vi "Plugin - Compute Turns.vi"(11 "Message Queues in":T1) -> ()   [LabVIEW 2019]
uses:
  support/Copy of Message Queue/All Message Queues.ctl
  support/Copy of Message Queue/Message Cluster.ctl
  support/Global Offsets.vi
  Acquisition/Acquisition.lvlib
  support/Message Queue/Message Queue.lvlib
  support/Copy of Message Queue/Copy of Message Queue.lvlib
panel:
  in  "OK":bool
  out "Turns Clockwise":dbl format="%.3f"
  in  "Stop":bool
  out "T12":dbl(slide) scale=0.0..30.0
  out "T11":dbl(slide) scale=0.0..30.0
  out "T10":dbl(slide) scale=0.0..30.0
  out "T9":dbl(slide) scale=0.0..30.0
  out "T8":dbl(slide) scale=0.0..30.0
  out "T7":dbl(slide) scale=0.0..30.0
  out "T6":dbl(slide) scale=0.0..30.0
  out "T5":dbl(slide) scale=0.0..30.0
  out "T4":dbl(slide) scale=0.0..30.0
  out "T3":dbl(slide) scale=0.0..30.0
  out "T2":dbl(slide) scale=0.0..30.0
  out "T1":dbl(slide) scale=0.0..30.0
  out "Aquatrak RS232 Output":string
  in  "error in":errorcluster
  out "error out":errorcluster
  # "Compute Turns Clockwise"
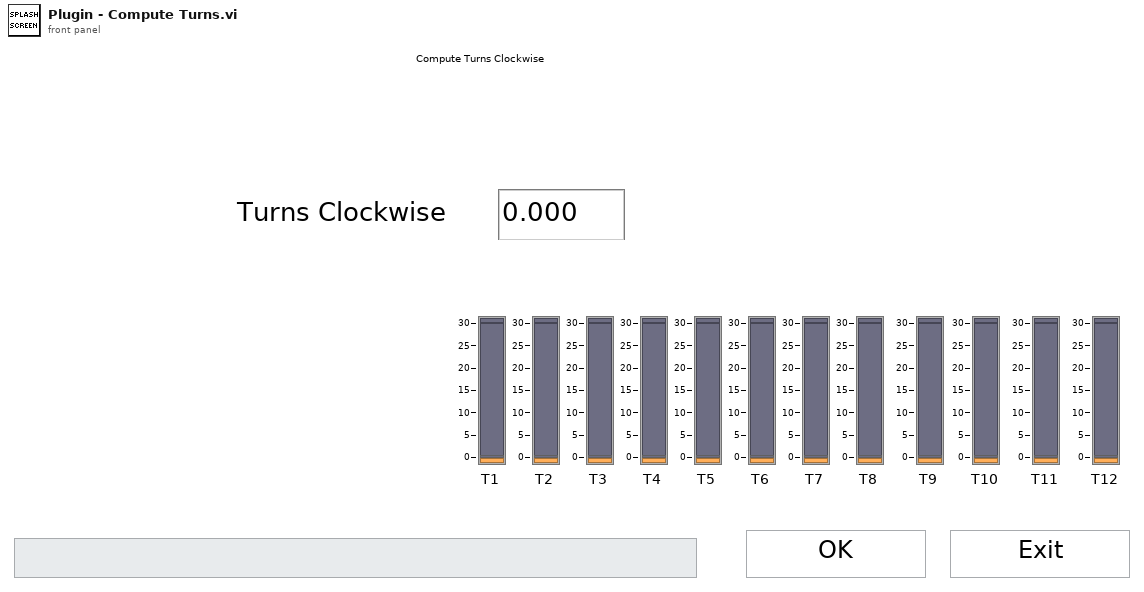
[diagram p1: front panel]
types:
  T1 = typedef "Copy of Message Queue.lvlib/All Message Queues.ctl" = cluster{"UI":refnum<queue>, "Acquisition":refnum<queue>, "Logging":refnum<queue>, "Analyze":refnum<queue>}
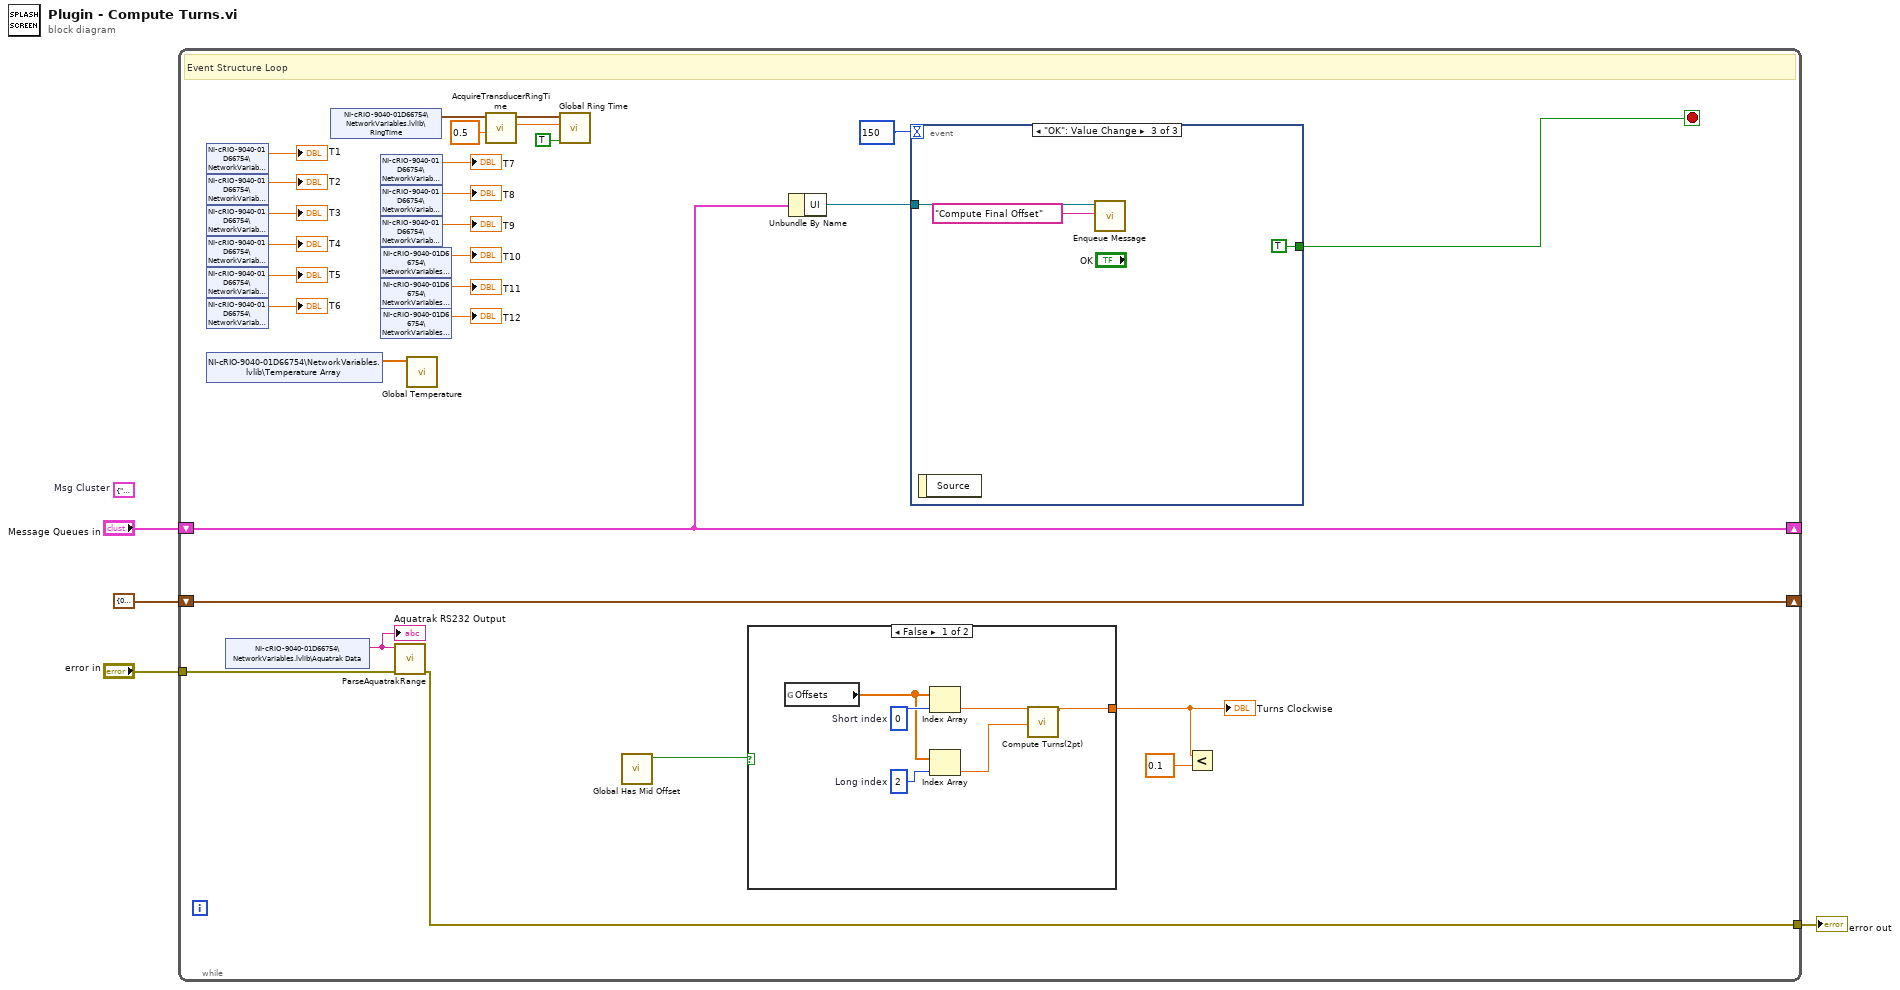
[diagram p0: block diagram]
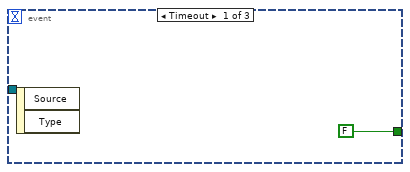
[diagram p2: hidden frame]
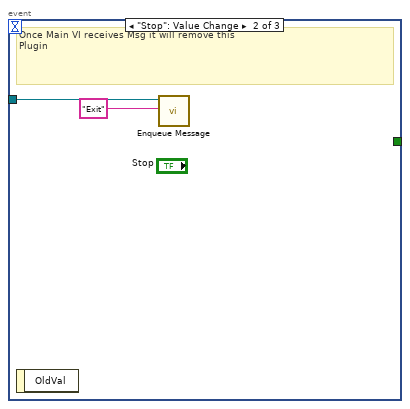
[diagram p3: hidden frame]
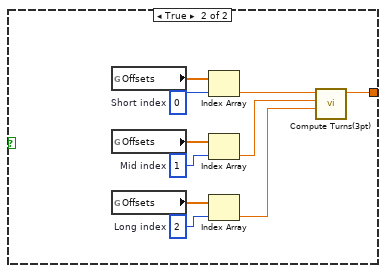
[diagram p4: hidden frame]
diagram:
  (unwired) cluster{"Msg":string, "Data":variant} {"Msg"="", "Data"=variant}  # Msg Cluster
  n1 = while {
    shift-right: [w12] -> _
    shift-left: "Message Queues in" -> [w12]
    shift-right: [w20] -> _
    shift-left: cluster{"Raw Offset":dbl, "Corr. Offset":dbl} {"Raw Offset"=0.0, "Corr. Offset"=0.0} -> [w20]
    tunnel: [w13] -> w2
    tunnel: "error in" -> [w14]
    stop <- w5 stop-if-true
    # "Event Structure Loop"
    n2 = shared-variable "NI-cRIO-9040-01D66754\\NetworkVariables.lvlib\\T1"() -> (→"T1":dbl)  [unwired: 1 in, 1 out]
    n3 = shared-variable "NI-cRIO-9040-01D66754\\NetworkVariables.lvlib\\T2"() -> (→"T2":dbl)  [unwired: 1 in, 1 out]
    n4 = shared-variable "NI-cRIO-9040-01D66754\\NetworkVariables.lvlib\\T3"() -> (→"T3":dbl)  [unwired: 1 in, 1 out]
    n5 = shared-variable "NI-cRIO-9040-01D66754\\NetworkVariables.lvlib\\T4"() -> (→"T4":dbl)  [unwired: 1 in, 1 out]
    n6 = shared-variable "NI-cRIO-9040-01D66754\\NetworkVariables.lvlib\\T5"() -> (→"T5":dbl)  [unwired: 1 in, 1 out]
    n7 = shared-variable "NI-cRIO-9040-01D66754\\NetworkVariables.lvlib\\T6"() -> (→"T6":dbl)  [unwired: 1 in, 1 out]
    n8 = shared-variable "NI-cRIO-9040-01D66754\\NetworkVariables.lvlib\\Temperature Array"() -> (w18:dbl[])  [unwired: 1 in, 1 out]
    n9 = shared-variable "NI-cRIO-9040-01D66754\\NetworkVariables.lvlib\\Aquatrak Data"() -> (w19:string)  [unwired: 1 in, 1 out]
    "Aquatrak RS232 Output" <- w19
    n10 = shared-variable "NI-cRIO-9040-01D66754\\NetworkVariables.lvlib\\RingTime"() -> (w33:waveform(dbl)[])  [unwired: 1 in, 1 out]
    n11 = shared-variable "NI-cRIO-9040-01D66754\\NetworkVariables.lvlib\\T7"() -> (→"T7":dbl)  [unwired: 1 in, 1 out]
    n12 = shared-variable "NI-cRIO-9040-01D66754\\NetworkVariables.lvlib\\T8"() -> (→"T8":dbl)  [unwired: 1 in, 1 out]
    n13 = shared-variable "NI-cRIO-9040-01D66754\\NetworkVariables.lvlib\\T9"() -> (→"T9":dbl)  [unwired: 1 in, 1 out]
    n14 = shared-variable "NI-cRIO-9040-01D66754\\NetworkVariables.lvlib\\T10"() -> (→"T10":dbl)  [unwired: 1 in, 1 out]
    n15 = shared-variable "NI-cRIO-9040-01D66754\\NetworkVariables.lvlib\\T11"() -> (→"T11":dbl)  [unwired: 1 in, 1 out]
    n16 = shared-variable "NI-cRIO-9040-01D66754\\NetworkVariables.lvlib\\T12"() -> (→"T12":dbl)  [unwired: 1 in, 1 out]
    n17 = call "ParseAquatrakRange.vi"("error in"=w14, "Incoming String"=w19) -> ("error out"=w13:errorcluster)  [unwired: 5 in, 4 out]
    n18 = call "Global Temperature.vi"("Temp In"=w18) -> ()  [unwired: 9 in, 2 out]
    n19 = call "AcquireTransducerRingTime.vi"("Cut-Off Level"=0.5, "Ring Time Wavefrom Array"=w33) -> ("Ring Time (ms)"=w16:dbl, "Ring Time Wavefrom"=w17:waveform(dbl))  [unwired: 7 in, 1 out]
    n20 = call "Global Ring Time.vi"("Ring Time Plot In"=w17, "Ring Time (ms) In"=w16, "Set Data?"=TRUE) -> ()  [unwired: 6 in, 2 out]
    n21 = call "Global Has Mid Offset.vi"() -> ("Has M Offset? out"=w10:bool)  [unwired: 10 in]
    n22 = case shown="False" w10 {
      tunnel: [w41 w46] -> w9
      frame False {
        w44 = 2  # Long index
        w45 = 0  # Short index
        n23 = global read "Global Offsets.vi" "Offsets"() -> (w40:dbl[])
        n24 = Index Array(array=w40, index=w45) -> (element=w43:dbl)
        n25 = Index Array(array=w40, index=w44) -> (element=w42:dbl)
        n26 = call "Compute Turns(2pt).vi"("Long Offset"=w42, "Short Offset"=w43) -> ("Turns Clockwise"=w41:dbl)  [unwired: 9 in]
      }
      frame True {
        w50 = 2  # Long index
        w51 = 1  # Mid index
        w54 = 0  # Short index
        n27 = global read "Global Offsets.vi" "Offsets"() -> (w55:dbl[])
        n28 = global read "Global Offsets.vi" "Offsets"() -> (w52:dbl[])
        n29 = global read "Global Offsets.vi" "Offsets"() -> (w49:dbl[])
        n30 = Index Array(array=w55, index=w54) -> (element=w53:dbl)
        n31 = Index Array(array=w52, index=w51) -> (element=w48:dbl)
        n32 = Index Array(array=w49, index=w50) -> (element=w47:dbl)
        n33 = call "Compute Turns(3pt).vi"("Long Offset"=w47, "Mid Offset"=w48, "Short Offset"=w53) -> ("Turns Clockwise"=w46:dbl)  [unwired: 8 in]
      }
    }
    "Turns Clockwise" <- w9
    n34 = Unbundle By Name(w12) -> ("UI"=w6:refnum<queue>)
    n35 = event shown="[2] \"OK\": Value Change" {
      selector: _ -> [_ _ _]
      dyn-events: _ -> [_ _ _]
      timeout: 150 -> [_ _ _]
      tunnel: w6 -> [_ w35 w38]
      tunnel: [FALSE _ TRUE] -> w5
      event Timeout {
        n36 = event-data() -> ()  [unwired: 1 in, 2 out]
      }
      event "Stop": Value Change {
        # "Once Main VI receives Msg it will remove this \nPlugin"
        n37 = event-data() -> ()  [unwired: 1 in, 1 out]
        n38 = call "Enqueue Message.vi"("Message"="Exit", "Message Queue"=w35) -> ()  [unwired: 8 in, 2 out]
      }
      event "OK": Value Change {
        n39 = event-data() -> ()  [unwired: 1 in, 1 out]
        n40 = call "Enqueue Message.vi"("Message"="Compute Final Offset", "Message Queue"=w38) -> ()  [unwired: 8 in, 2 out]
      }
    }
    n41 = Less?(x=w9, y=0.1 ("Turns Clockwise")) -> ()  [unwired: 1 out]
  }
  "error out" <- w2
